vi "Timer_ISR.vi"(11 "TIMX_Interrupt":T1) -> ()   [LabVIEW 2011]
uses:
  D:/National Instruments/LabVIEW 2011/Targets/Keil/Embedded/RealView/Generic/My_ARM_Starter_Board_F4/STM32_DriverVI_Interface/Timer/Timer_ISR_F4.ctl
  <vilib>/eio/EIO_TerminalDirection.ctl
  <vilib>/STM32_DriverVI_Interface_F4/GPIO_EIO/GPO_EIO_Inner_F4.vi
  <vilib>/eio/EIONode/EIONode.xnode
panel:
  # "这是一个标准的中断模板 VI，用户可以直接使用,\n在相应的Case语句里面实现相应的中断服务程序即可！\n\n双击打开这个VI之后，另存为副本，名称不变，将其保存\n并添加到项目浏览器中，然后在程序生成规范中进行属性\n设置！"
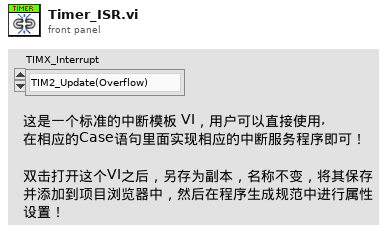
[diagram p1: front panel]
types:
  T1 = typedef "Timer_ISR_F4.ctl" = enum8{"TIM2_Update(Overflow)", "TIM2_Channel_1", "TIM2_Channel_2", "TIM2_Channel_3", "TIM2_Channel_4", "TIM3_Update(Overflow)", "TIM3_Channel_1", "TIM3_Channel_2", "TIM3_Channel_3", "TIM3_Channel_4", "TIM4_Update(Overflow)", "TIM4_Channel_1", "TIM4_Channel_2", "TIM4_Channel_3", "TIM4_Channel_4", "TIM5_Update(Overflow)", "TIM5_Channel_1", "TIM5_Channel_2", "TIM5_Channel_3", "TIM5_Channel_4", "TIM6_Update(Overflow)", "TIM7_Update(Overflow)", "----------------------------", "WWDG_ISR", "RTC_Alarm_ClockA_ISR", "RTC_Alarm_ClockB_ISR", "RTC_WKUP_ISR", "TIM1_Update(Overflow)", "TIM1_Channel_1", "TIM1_Channel_2", "TIM1_Channel_3", "TIM1_Channel_4", "TIM8_Update(Overflow)", "TIM8_Channel_1", "TIM8_Channel_2", "TIM8_Channel_3", "TIM8_Channel_4", "TIM9_Update(Overflow)", "TIM9_Channel_1", "TIM9_Channel_2", "TIM10_Update(Overflow)", "TIM10_Channel_1", "TIM11_Update(Overflow)", "TIM11_Channel_1", "TIM12_Update(Overflow)", "TIM12_Channel_1", "TIM12_Channel_2", "TIM13_Update(Overflow)", "TIM13_Channel_1", "TIM14_Update(Overflow)", "TIM14_Channel_1"}
  T2 = enum8{"P0", "P1", "P2", "P3", "P4", "P5", "P6", "P7", "P8", "P9", "P10", "P11", "P12", "P13", "P14", "P15"}
  T3 = typedef "RTC中断类型_F4.ctl" = enum8{"Alarm A Interrupt", "Alarm B Interrupt", "RTC WKUP（Overflow） Int"}
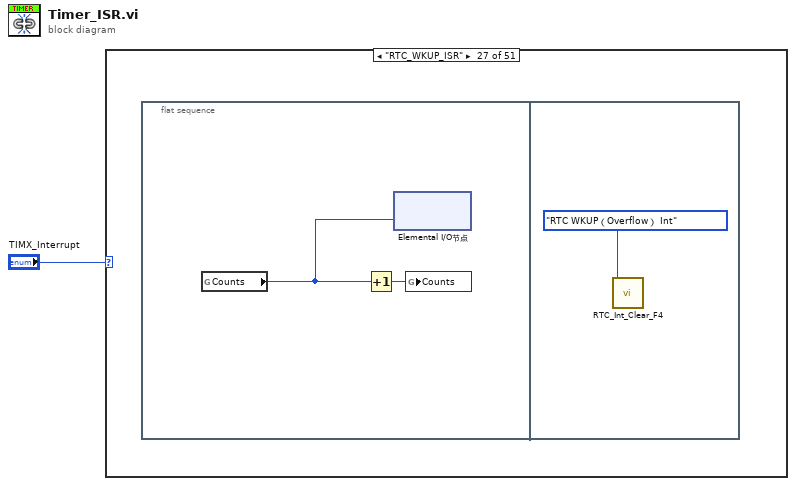
[diagram p0: block diagram]
diagram:
  n1 = case shown="\"RTC_WKUP_ISR\"" "TIMX_Interrupt" {
    frame "TIM2_Update(Overflow)", Default {
      n2 = flat-sequence {
        frame #0 {
          # "更新中断服务程序"
        }
        frame #1 {
          # "清除更新中断标志位"
        }
      }
    }
    frame "TIM2_Channel_1" {
    }
    frame "TIM2_Channel_2" {
      # "一个中断号只对应一个引脚中断时，直接处理"
    }
    frame "TIM2_Channel_3" {
    }
    frame "TIM2_Channel_4" {
    }
    frame "TIM3_Update(Overflow)" {
    }
    frame "TIM3_Channel_1" {
    }
    frame "TIM3_Channel_2" {
    }
    frame "TIM3_Channel_3" {
    }
    frame "TIM3_Channel_4" {
    }
    frame "TIM4_Update(Overflow)" {
    }
    frame "TIM4_Channel_1" {
    }
    frame "TIM4_Channel_2" {
    }
    frame "TIM4_Channel_3" {
    }
    frame "TIM4_Channel_4" {
    }
    frame "TIM5_Update(Overflow)" {
    }
    frame "TIM5_Channel_1" {
    }
    frame "TIM5_Channel_2" {
    }
    frame "TIM5_Channel_3" {
    }
    frame "TIM5_Channel_4" {
    }
    frame "TIM6_Update(Overflow)" {
    }
    frame "TIM7_Update(Overflow)" {
    }
    frame "----------------------------" {
    }
    frame "WWDG_ISR" {
    }
    frame "RTC_Alarm_ClockA_ISR" {
    }
    frame "RTC_Alarm_ClockB_ISR" {
    }
    frame "RTC_WKUP_ISR" {
      n3 = flat-sequence {
        frame #0 {
          n4 = global read "全局变量.vi" "Counts"() -> (w2:u16)
          n5 = Increment(x=w2) -> (x+1=w3:u16)
          n6 = xnode "Elemental I/O节点"("LED_1"=w2) -> ()  [unwired: 1 in, 1 out]
          n7 = global write "全局变量.vi" "Counts"(w3) -> ()
        }
        frame #1 {
          n8 = call <vilib>:"RTC_Int_Clear_F4.vi"("RTC中断标志位"=RTC中断类型_F4."RTC WKUP（Overflow） Int") -> ()  [unwired: 10 in, 1 out]
        }
      }
    }
    frame "TIM1_Update(Overflow)" {
    }
    frame "TIM1_Channel_1" {
    }
    frame "TIM1_Channel_2" {
    }
    frame "TIM1_Channel_3" {
    }
    frame "TIM1_Channel_4" {
    }
    frame "TIM8_Update(Overflow)" {
    }
    frame "TIM8_Channel_1" {
    }
    frame "TIM8_Channel_2" {
    }
    frame "TIM8_Channel_3" {
    }
    frame "TIM8_Channel_4" {
    }
    frame "TIM9_Update(Overflow)" {
    }
    frame "TIM9_Channel_1" {
    }
    frame "TIM9_Channel_2" {
    }
    frame "TIM10_Update(Overflow)" {
    }
    frame "TIM10_Channel_1" {
    }
    frame "TIM11_Update(Overflow)" {
    }
    frame "TIM11_Channel_1" {
    }
    frame "TIM12_Update(Overflow)" {
    }
    frame "TIM12_Channel_1" {
    }
    frame "TIM12_Channel_2" {
    }
    frame "TIM13_Update(Overflow)" {
    }
    frame "TIM13_Channel_1" {
    }
    frame "TIM14_Update(Overflow)" {
    }
    frame "TIM14_Channel_1" {
    }
  }
